vi "mc_run_sequence (SubVI).vi"(1 "Basler COM":refnum<visa-resource-name>, 5 "Arduino Digital \nOutput Channel":u8=13, 7 "Array":cluster{dbl, dbl, dbl}[](array[cluster]), 8 "Number of Cycles":i32=1, 9 "Time Between Cycles (s)":dbl, 10 "error in (no error)":errorcluster, 11 ".NET Refnum in":refnum<k24>) -> (0 "Current Z":dbl, 2 "error out":errorcluster, 3 ".NET Refnum out":refnum<k24>, 4 "Current Y":dbl, 6 "Current X":dbl)   [LabVIEW 2026]
uses:
  C:/Program Files (x86)/Control/SC3U.dll
  Program Files (x86)/Control/SC3U.dll
  <vilib>/MakerHub/LINX/Public/Utilities/Open Serial.vi
  <vilib>/MakerHub/LINX/LMH-LINX.lvlib
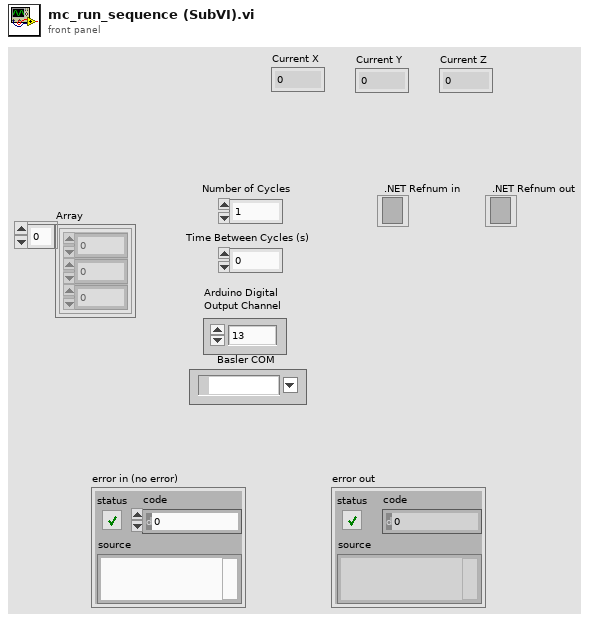
[diagram p1: front panel]
types:
  T1 = typedef "LMH-LINX.lvlib/LINX Ref.ctl" = cluster{"IO":T2, "Interface":T3, "LINX Device Config":T4}
  T2 = typedef "LMH-LINX.lvlib/Platform.ctl" = enum16{"Remote", "Local"}
  T3 = typedef "LMH-LINX.lvlib/Interface.ctl" = enum16{"Serial", "TCP"}
  T4 = typedef "LMH-LINX.lvlib/Device.lvlib/LINX Device Config.ctl" = cluster{"Interface":T3, "COM Port":refnum<visa-resource-name>, "TCP Configuration":T5, "Device Family":u8, "Device ID":u8, "Device Name":string, "TCP Ref":refnum<k5>, "Channels":T6}
  T5 = typedef "LMH-LINX.lvlib/Device.lvlib/TCP Config.ctl" = cluster{"IP Address":string, "Port":u16}
  T6 = typedef "LMH-LINX.lvlib/Channels.ctl" = cluster{"DI":u8[], "DO":u8[], "AI":u8[], "AO":u8[], "PWM":u8[], "QE":u8[], "UART":u8[], "I2C 2":u8[], "SPI":u8[], "CAN":u8[], "Servo":u8[], "AI Ref (V)":dbl, "AI Resolution (Bits)":u8, "AO Ref (V)":dbl, "AO Resolution (Bits)":u8}
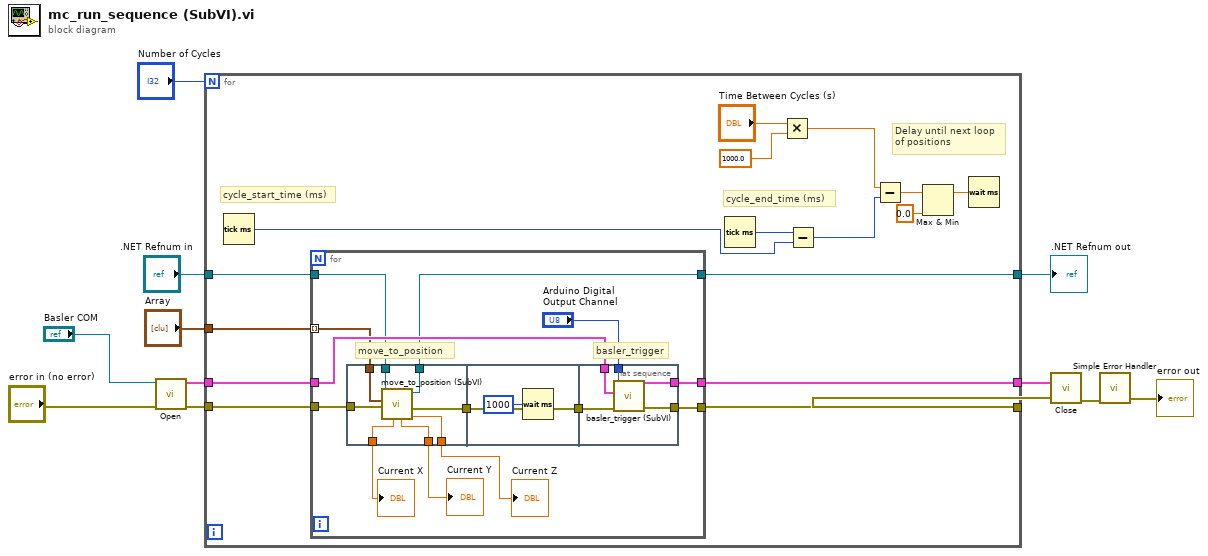
[diagram p0: block diagram]
diagram:
  n1 = call-poly <vilib>:"Open.vi"("Error In"="error in (no error)", "Serial Port"="Basler COM") -> ("Error Out"=w9:errorcluster, "LINX Resource"=w8:T1)  [unwired: 7 in, 1 out]
  n2 = for {
    N: "Number of Cycles" -> [_]
    tunnel: "Array" -> [w28]
    tunnel: [w27] -> w12
    tunnel: ".NET Refnum in" -> [w26]
    tunnel: w9 -> [w25]
    tunnel: w8 -> [w24]
    tunnel: [w23] -> w6
    tunnel: [w22] -> w5
    # "Delay until next loop of positions"
    # "cycle_end_time (ms)"
    # "cycle_start_time (ms)"
    n3 = Tick Count (ms)() -> (millisecond timer value=w20:u32)
    n4 = for {
      tunnel: w28 -> [w36] mode=indexing
      tunnel: [w33] -> w27
      tunnel: w26 -> [w35]
      tunnel: w25 -> [w37]
      tunnel: w24 -> [w41]
      tunnel: [w39] -> w23
      tunnel: [w38] -> w22
      # "basler_trigger"
      # "move_to_position"
      n5 = flat-sequence {
        tunnel: w37 -> [w49]
        tunnel: w36 -> [w48]
        tunnel: w35 -> [w47]
        tunnel: [w46] -> w34
        tunnel: [w45] -> w33
        tunnel: [w44] -> w32
        tunnel: [w43] -> w31
        tunnel: [w42] -> w30
        tunnel: w30 -> [w50]
        tunnel: [w50] -> w29
        tunnel: w41 -> [w56]
        tunnel: "Arduino Digital \nOutput Channel" -> [w55]
        tunnel: [w54] -> w39
        tunnel: [w53] -> w38
        tunnel: w29 -> [w52]
        frame #0 {
          n6 = call "move_to_position (SubVI).vi"("error in (no error)"=w49, "Cluster"=w48, ".NET Refnum in"=w47) -> ("Current Z"=w46:dbl, "error out"=w42:errorcluster, ".NET Refnum out"=w45:refnum<k24>, "Current Y"=w44:dbl, "Current X"=w43:dbl)  [unwired: 4 in]
        }
        frame #1 {
          n7 = Wait (ms)(milliseconds to wait=u32 1000) -> ()  [unwired: 1 out]
        }
        frame #2 {
          n8 = call "basler_trigger (SubVI).vi"("error in (no error)"=w52, "LINX Resource in"=w56, "Arduino Digital \nOutput Channel"=w55) -> ("error out"=w54:errorcluster, "LINX Resource out"=w53:T1)  [unwired: 7 in]
        }
      }
      "Current X" <- w31
      "Current Z" <- w34
      "Current Y" <- w32
    }
    n9 = Tick Count (ms)() -> (millisecond timer value=w21:u32)
    n10 = Multiply(x="Time Between Cycles (s)", y=1000.0) -> (x*y=w17:dbl)
    n11 = Subtract(x=w21, y=w20) -> (x-y=w16:u32)
    n12 = Subtract(x=w17, y=w16) -> (x-y=w15:dbl)
    n13 = Max & Min(x=w15, y=0.0) -> (max(x,y)=w13:dbl)  [unwired: 1 out]
    n14 = Wait (ms)(milliseconds to wait=w13) -> ()  [unwired: 1 out]
  }
  ".NET Refnum out" <- w12
  n15 = call <vilib>:"Close.vi"("Error In"=w6, "LINX Resource"=w5) -> ("Error Out"=w4:errorcluster)  [unwired: 9 in]
  n16 = call <vilib>:"Simple Error Handler.vi"("error in (no error)"=w4) -> ("error out"=→"error out":errorcluster)  [unwired: 4 in, 4 out]
